vi "Main.vi"() -> ()   [LabVIEW 2017, in "Settings Editor.lvlib"]
doc: "This template is based off of the Queued Message Handler design pattern and the Queued Message Handler project template that ships with LabVIEW.\n\nThe main difference is that the queue is private to this module and communication between modules is performed via Broadcast and Request events.\n\nRequest events are wrapped in public API methods and are handled in the Event Handling Loop (EHL) of this VI. Any module can register for Broadcast events sent by this module. The EHL generates messages based on user interface actions.\n\nThe Message Handling Loop (MHL) processes messages generated by the EHL, or by other messages. The messages are string values, so new messages can be added easily to the Message Cases case structure in the MHL. Each message cluster can also provide an optional value for Message Data, which is a variant that can be converted to whatever message-specific data is required.\n_____\nBased on Delacor QMH Project Template 4.0.0.47.\n_____\nBased on Delacor QMH Project Template 4.1.0.56."
uses:
  Settings Editor.lvlib
  <vilib>/Delacor/Delacor QMH/Libraries/Module Admin_class/Delacor_lib_QMH_Module Admin.lvclass
  CML Shared/Signal Type--enum.ctl
  CML Shared/Calibration Values--cluster.ctl
  Module Data--cluster.ctl
  Settings--cluster.ctl
  Stop Argument--cluster.ctl
  Update Application Settings Argument--cluster.ctl
  Update Application Settings (Reply Payload)--cluster.ctl
  <vilib>/Delacor/Delacor QMH/Libraries/Module Admin_class/Delacor_lib_QMH_Module Admin.lvclass/Delacor_lib_QMH_Module Admin.ctl
  <vilib>/Utility/miscctls.llb/LVPointTypeDef.ctl
  <vilib>/Delacor/Delacor QMH/Libraries/Module Admin_class/Delacor_lib_QMH_Get External Launch.vi
  <vilib>/Delacor/Delacor QMH/Libraries/Message Queue_class/Delacor_lib_QMH_Enqueue Message (Single).vi
  <vilib>/Utility/error.llb/Error Cluster From Error Code.vi
  <vilib>/ErrorRing/Error Ring.xnode
  <vilib>/Delacor/Delacor QMH/Libraries/Message Queue_class/Delacor_lib_QMH_Message Queue.lvclass
  CML Shared/CML Shared.lvlib
panel:
  in  "Calibration Values":T1[](array[typedef])
  in  "Cancel":bool
  in  "OK":bool
  in  "Log File Base Path":path
  in  "Signal Type":T2
  out "error out":errorcluster
  in  "Module Admin":refnum<class "Delacor_lib_QMH_Module Admin.lvclass">
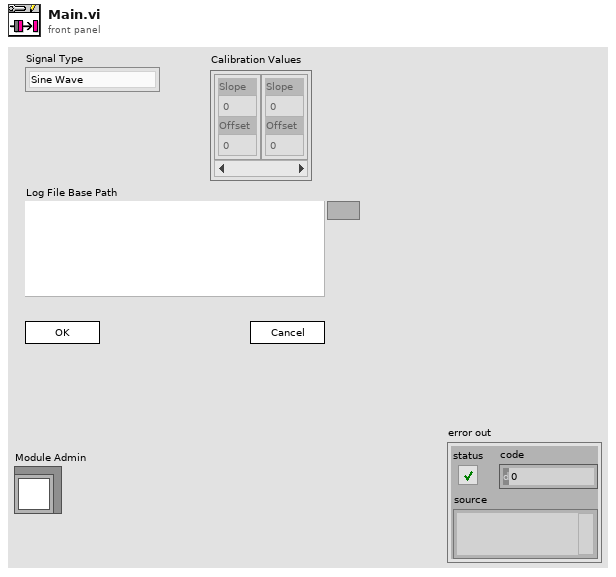
[diagram p1: front panel]
types:
  T1 = typedef "CML Shared.lvlib/Calibration Values--cluster.ctl" = cluster{"Slope":dbl, "Offset":dbl}
  T2 = typedef "CML Shared.lvlib/Signal Type--enum.ctl" = enum16{"Sine Wave", "Square with Noise"}
  T3 = typedef "Settings Editor.lvlib/Request Events--cluster.ctl" = cluster{"Stop Module":refnum<user-event>, "Show Panel":refnum<user-event>, "Hide Panel":refnum<user-event>, "Get Module Execution Status":refnum<user-event>, "Show Diagram":refnum<user-event>, "Update Application Settings":refnum<user-event>}
  T4 = typedef "Settings Editor.lvlib/Module Data--cluster.ctl" = cluster{"Settings":T5}
  T5 = typedef "Settings Editor.lvlib/Settings--cluster.ctl" = cluster{"Signal Type":T2, "Calibration Array":T1[], "Log File Base Path":path}
  T6 = enum32{"invalid lock state", "Not Locked", "Locked (No Password)", "Password-protected"}
  T7 = typedef "Settings Editor.lvlib/Stop Argument--cluster.ctl" = cluster{"Origin":string, "Exit via Stop Module Req?":bool, "Wait for Module to stop?":bool}
  T8 = typedef "Settings Editor.lvlib/Update Application Settings Argument--cluster.ctl" = cluster{"Wait Notifier":refnum<notifier>, "wait for reply":bool}
  T9 = typedef "LVPointTypeDef.ctl" = cluster{"Horizontal":i16, "Vertical":i16}
  T10 = enum32{"Invalid", "Standard", "Closed", "Hidden", "Minimized", "Maximized"}
  T11 = typedef "Settings Editor.lvlib/Update Application Settings (Reply Payload)--cluster.ctl" = cluster{"Settings":T5, "Update Settings_error":errorcluster}
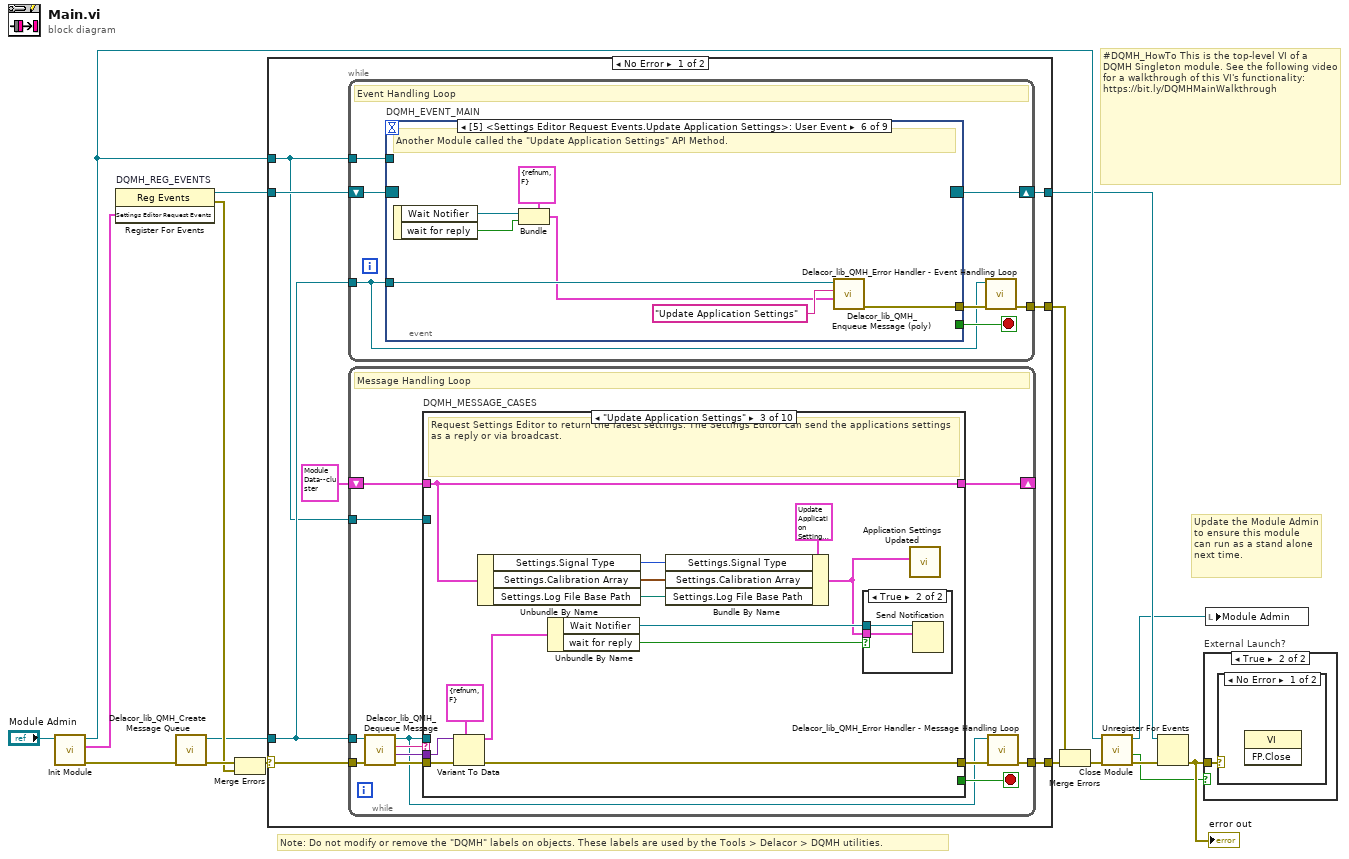
[diagram p0: block diagram]
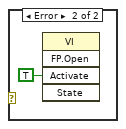
[diagram p3: hidden frame]
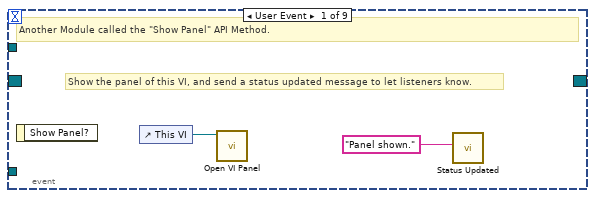
[diagram p4: hidden frame]
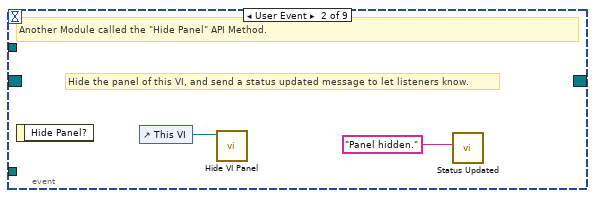
[diagram p5: hidden frame]
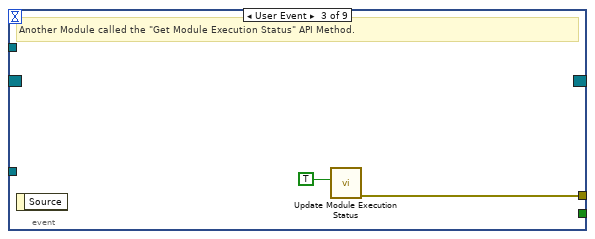
[diagram p6: hidden frame]
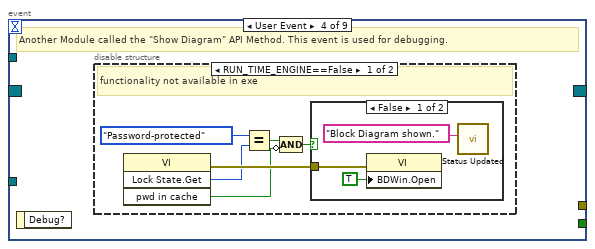
[diagram p7: hidden frame]
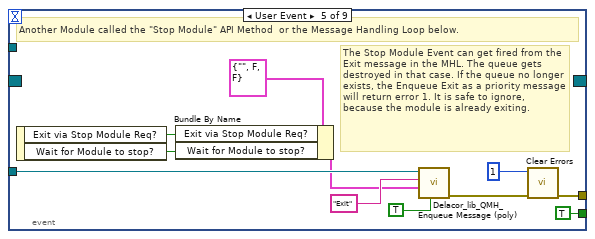
[diagram p10: hidden frame]
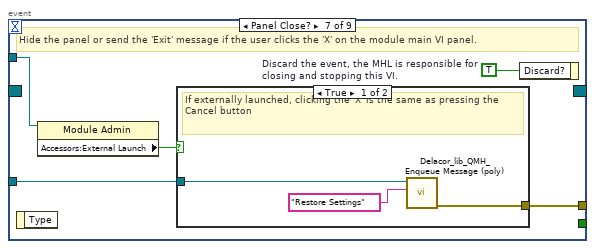
[diagram p11: hidden frame]
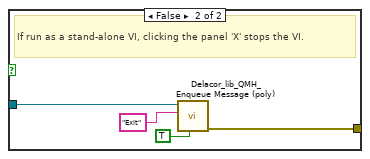
[diagram p12: hidden frame]
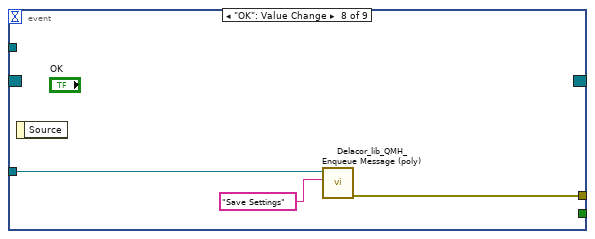
[diagram p13: hidden frame]
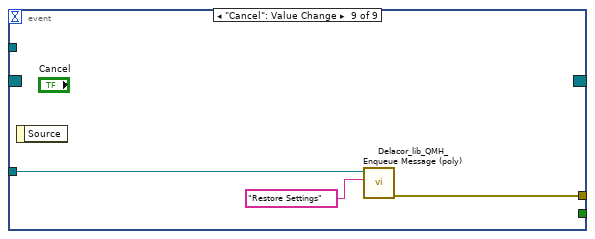
[diagram p14: hidden frame]
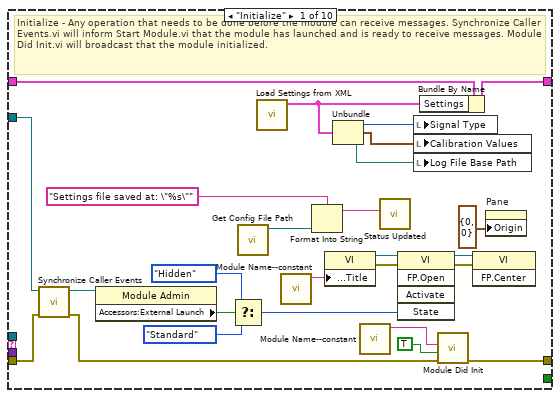
[diagram p15: hidden frame]
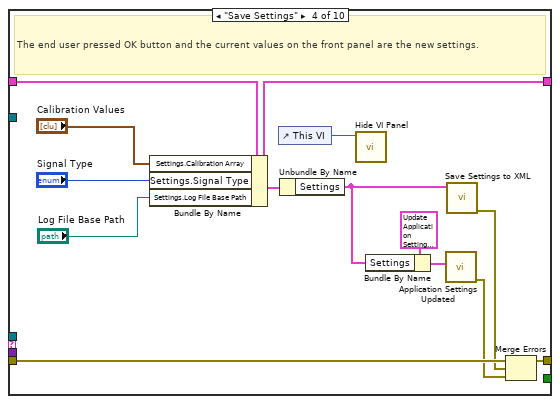
[diagram p18: hidden frame]
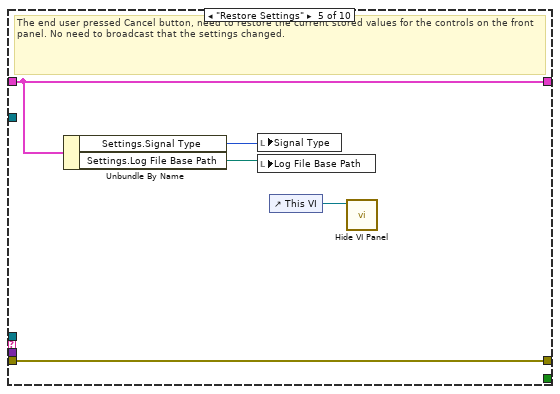
[diagram p19: hidden frame]
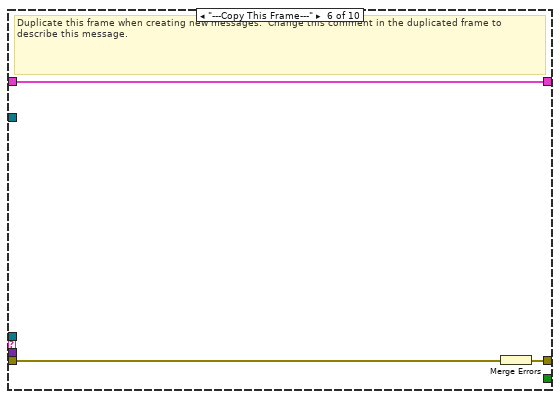
[diagram p20: hidden frame]
diagram:
  # "#DQMH_HowTo This is the top-level VI of a DQMH Singleton module. See the following video for a walkthrough of this VI's functionality: https://bit.ly/DQMHMainWalkthrough"
  # "Note: Do not modify or remove the \"DQMH\" labels on objects. These labels are used by the Tools > Delacor > DQMH utilities."
  # "Update the Module Admin to ensure this module can run as a stand alone next time."
  n1 = call "Init Module.vi"("Singleton Module Admin in"="Module Admin") -> ("error out"=w16:errorcluster, "Settings Editor Request Events"=w5:T3, "Singleton Module Admin out"=w8:refnum<class "Delacor_lib_QMH_Module Admin.lvclass">)  [unwired: 8 in]
  n2 = register-events "DQMH_REG_EVENTS"(w5) -> (reference out=w6:refnum<event-registration>, error out=w9:errorcluster)  [unwired: 2 in]
  n3 = call <vilib>:"Delacor_lib_QMH_Create Message Queue.vi"("error in (no error)"=w16) -> ("error out"=w11:errorcluster, "Message Queue"=w4:refnum<class "Delacor_lib_QMH_Message Queue.lvclass">)  [unwired: 9 in]
  n4 = Merge Errors(w11, w9) -> (w10:errorcluster)
  n5 = case shown="No Error" w10 {
    selector: w10 -> [w23 w214]
    tunnel: [w25 w214] -> w17
    tunnel: [w22 w211] -> w7
    tunnel: w6 -> [w20 w211]
    tunnel: w4 -> [w19 _]
    tunnel: [w24 _] -> w14
    tunnel: w8 -> [w18 w207]
    frame No Error {
      n6 = while {
        tunnel: w19 -> [w26]
        shift-right: [w29] -> w22
        shift-left: w20 -> [w30]
        tunnel: [w31] -> w24
        tunnel: w18 -> [w27]
        stop <- w28 stop-if-true
        # "Event Handling Loop"
        n7 = event "DQMH_EVENT_MAIN" shown="[5] <Settings Editor Request Events.Update Application Settings>: User Event" {
          selector: w30 -> [_ _ _ _ _ _ _ _ _]
          dyn-events: [_ _ _ _ _ _ _ _ _] -> w29
          timeout: _ -> [_ _ _ _ _ _ _ _ _]
          tunnel: [_ _ _ _ TRUE ("Discard?") _ _ _ _] -> w28
          tunnel: w26 -> [_ _ _ _ w54 w65 w68 w78 w82]
          tunnel: [_ _ w38 _ w57 w61 w70 w79 w81] -> w32
          tunnel: w27 -> [_ _ _ _ _ _ w67 _ _]
          event User Event {
            # "Show the panel of this VI, and send a status updated message to let listeners know."
            # "Another Module called the \"Show Panel\" API Method."
            n8 = event-data() -> ()  [unwired: 1 in, 1 out]
            n9 = control-ref of="This VI"() -> (w34:refnum<vi>)
            n10 = call "Open VI Panel.vi"("VI"=w34) -> ()  [unwired: 10 in, 1 out]
            n11 = call "Status Updated.vi"("Status"="Panel shown." ("format string")) -> ()  [unwired: 10 in, 1 out]
          }
          event User Event {
            # "Hide the panel of this VI, and send a status updated message to let listeners know."
            # "Another Module called the \"Hide Panel\" API Method."
            n12 = event-data() -> ()  [unwired: 1 in, 1 out]
            n13 = control-ref of="This VI"() -> (w36:refnum<vi>)
            n14 = call "Hide VI Panel.vi"("VI"=w36) -> ()  [unwired: 10 in, 1 out]
            n15 = call "Status Updated.vi"("Status"="Panel hidden." ("format string")) -> ()  [unwired: 10 in, 1 out]
          }
          event User Event {
            # "Another Module called the \"Get Module Execution Status\" API Method."
            n16 = event-data() -> ()  [unwired: 1 in, 1 out]
            n17 = call "Update Module Execution Status.vi"("Running?"=TRUE) -> ("error out"=w38:errorcluster)  [unwired: 10 in]
          }
          event User Event {
            # "Another Module called the \"Show Diagram\" API Method. This event is used for debugging."
            n18 = event-data() -> ()  [unwired: 1 in, 1 out]
            n19 = disable-structure shown="RUN_TIME_ENGINE==False" {
              frame condition #0 (active) {
                # "functionality not available in exe"
                n20 = invoke class="VI" method="Lock State.Get"() -> (error out=w44:errorcluster, "Get Lock State"=w43:T6, "pwd in cache"=w40:bool)  [unwired: 4 in, 1 out]
                n21 = Equal?(x=T6."Password-protected", y=w43) -> (x = y?=w41:bool)
                n22 = Compound Arithmetic op=AND(w41, invert w40) -> (w39:bool)
                n23 = case shown="False" w39 {
                  tunnel: w44 -> [w47 _]
                  frame False {
                    n24 = property class="VI"(error in=w47, "BDWin.Open"=TRUE ("Block Diagram Window:Open")) -> ()  [unwired: 1 in, 2 out]
                    n25 = call "Status Updated.vi"("Status"="Block Diagram shown." ("format string")) -> ()  [unwired: 10 in, 1 out]
                  }
                  frame True {
                    # "Password-protected VI, and the password is not in the cache. Do not show the diagram."
                  }
                }
              }
              frame condition #1 {
              }
            }
          }
          event User Event {
            # "The Stop Module Event can get fired from the Exit message in the MHL. The queue gets destroyed in that case. If the queue no longer exists, the Enqueue Exit as a priority message will return error 1. It is safe to ignore, because the module is already exiting."
            # "Another Module called the \"Stop Module\" API Method  or the Message Handling Loop below."
            n26 = event-data() -> ("Exit via Stop Module Req?"=w50:bool, "Wait for Module to stop?"=w49:bool)  [unwired: 1 in]
            n27 = Bundle By Name(cluster=T7 {"Origin"="", "Exit via Stop Module Req?"=FALSE, "Wait for Module to stop?"=FALSE} ("Stop Argument"), "Exit via Stop Module Req?"=w50, "Wait for Module to stop?"=w49) -> (w48:T7)
            n28 = call-poly <vilib>:"Delacor_lib_QMH_Enqueue Message (poly).vi"("Priority Message? (F)"=TRUE, "Message Data"=w48, "Message"="Exit", "Message Queue in"=w54) -> ("error out"=w58:errorcluster)  [unwired: 6 in, 1 out]
            n29 = call <vilib>:"Clear Errors.vi"("error in (no error)"=w58, "specific error code to clear (0: all)"=1) -> ("error out"=w57:errorcluster)  [unwired: 4 in, 1 out]
          }
          event User Event {
            # "Another Module called the \"Update Application Settings\" API Method."
            n30 = event-data() -> ("Wait Notifier"=w60:refnum<notifier>, "wait for reply"=w59:bool)  [unwired: 1 in]
            n31 = Bundle(cluster=T8 {"Wait Notifier"=refnum, "wait for reply"=FALSE} ("Update Application Settings Argument"), "Wait Notifier"=w60, "wait for reply"=w59) -> (w62:T8)
            n32 = call-poly <vilib>:"Delacor_lib_QMH_Enqueue Message (poly).vi"("Message Data"=w62, "Message"="Update Application Settings", "Message Queue in"=w65) -> ("error out"=w61:errorcluster)  [unwired: 7 in, 1 out]
          }
          event Panel Close? {
            w69 = TRUE  # Discard the event, the MHL is responsible for closing and stopping this VI.
            # "Hide the panel or send the 'Exit' message if the user clicks the 'X' on the module main VI panel."
            n33 = event-data() -> ()  [unwired: 1 in, 1 out]
            n34 = property class="Module Admin"(reference=w67) -> ("Accessors:External Launch"=w66:bool)  [unwired: 1 in, 2 out]
            n35 = case shown="True" w66 {
              tunnel: w68 -> [w72 w76]
              tunnel: [w71 w77] -> w70
              frame True {
                # "If externally launched, clicking the 'X' is the same as pressing the Cancel button"
                n36 = call-poly <vilib>:"Delacor_lib_QMH_Enqueue Message (poly).vi"("Message"="Restore Settings", "Message Queue in"=w72) -> ("error out"=w71:errorcluster)  [unwired: 8 in, 1 out]
              }
              frame False {
                # "If run as a stand-alone VI, clicking the panel 'X' stops the VI."
                n37 = call-poly <vilib>:"Delacor_lib_QMH_Enqueue Message (poly).vi"("Priority Message? (F)"=TRUE, "Message"="Exit", "Message Queue in"=w76) -> ("error out"=w77:errorcluster)  [unwired: 7 in, 1 out]
              }
            }
            n38 = event-data("Discard?"=w69) -> ()  [unwired: 1 in, 1 out]
          }
          event "OK": Value Change {
            n39 = event-data() -> ()  [unwired: 1 in, 1 out]
            n40 = call-poly <vilib>:"Delacor_lib_QMH_Enqueue Message (poly).vi"("Message"="Save Settings", "Message Queue in"=w78) -> ("error out"=w79:errorcluster)  [unwired: 8 in, 1 out]
          }
          event "Cancel": Value Change {
            n41 = event-data() -> ()  [unwired: 1 in, 1 out]
            n42 = call-poly <vilib>:"Delacor_lib_QMH_Enqueue Message (poly).vi"("Message"="Restore Settings", "Message Queue in"=w82) -> ("error out"=w81:errorcluster)  [unwired: 8 in, 1 out]
          }
        }
        n43 = call-dynamic "Delacor_lib_QMH_Error Handler - Event Handling Loop.vi"("error in (no error)"=w32, "Message Queue in"=w26) -> ("dup error in"=w31:errorcluster)  [unwired: 8 in, 1 out]
      }
      n44 = while {
        tunnel: w19 -> [w86]
        shift-right: [w90] -> _
        shift-left: T4 {"Settings"={"Signal Type"=enum."Sine Wave", "Calibration Array"=[{"Slope"=1.0, "Offset"=0.0}], "Log File Base Path"=path ""}} ("Data Cluster") -> [w91]
        tunnel: w23 -> [w94]
        tunnel: [w92] -> w25
        tunnel: w18 -> [w84]
        stop <- w89 stop-if-true
        # "Message Handling Loop"
        n45 = call-dynamic "Delacor_lib_QMH_Dequeue Message.vi"("error in (no error)"=w94, "Message Queue in"=w86) -> ("error out"=w93:errorcluster, "Message Data"=w87:variant, "Message"=w88:string, "Message Queue out"=w85:refnum<class "Delacor_lib_QMH_Message Queue.lvclass">)  [unwired: 6 in]
        n46 = case "DQMH_MESSAGE_CASES" shown="\"Update Application Settings\"" w88 {
          selector: w88 -> [_ _ _ _ _ _ _ _ _ w194]
          tunnel: w85 -> [_ _ _ _ _ _ _ w164 w186 _]
          tunnel: w93 -> [w120 w123 w136 w141 w156 w159 w161 w171 w192 w196]
          tunnel: [w118 w123 w135 w142 w156 w158 w161 w167 w189 w197] -> w95
          tunnel: w91 -> [w109 w122 w129 w151 w155 w157 w160 w166 w185 w195]
          tunnel: [w108 w122 w129 w148 w155 w157 w160 w166 w185 w195] -> w90
          tunnel: [_ _ _ _ _ _ _ _ w184 _] -> w89
          tunnel: w87 -> [_ _ w134 _ _ _ _ w165 w183 _]
          tunnel: w84 -> [w110 _ _ _ _ _ _ w163 w178 _]
          frame "Initialize" {
            # "Initialize - Any operation that needs to be done before the module can receive messages. Synchronize Caller Events.vi will inform Start Module.vi that the module has launched and is ready to receive messages. Module Did Init.vi will broadcast that the module initialized."
            n47 = call "Synchronize Caller Events.vi"("error in (no error)"=w120, "Singleton Module Admin in"=w110) -> ("error out"=w119:errorcluster, "Singleton Module Admin out"=w105:refnum<class "Delacor_lib_QMH_Module Admin.lvclass">)  [unwired: 8 in]
            n48 = property class="Module Admin"(reference=w105) -> ("Accessors:External Launch"=w114:bool)  [unwired: 1 in, 2 out]
            n49 = Select(t=T10."Hidden" ("State"), s=w114, f=T10."Standard" ("State")) -> (s? t:f=w111:T10)
            n50 = call "Get Config File Path.vi"() -> ("XML File Path"=w102:path)  [unwired: 10 in, 1 out]
            n51 = call "Load Settings from XML.vi"() -> ("Settings out"=w99:T5)  [unwired: 10 in, 1 out]
            n52 = call "Module Name--constant.vi"() -> ("Module Name"=w117:string)  [unwired: 11 in]
            n53 = Format Into String(format string="Settings file saved at: \"%s\"", w102) -> (resulting string=w101:string)  [unwired: 2 in, 1 out]
            n54 = property class="VI"("Front Panel.Title"=w117) -> (reference out=w116:refnum<vi>, error out=w103:errorcluster)  [unwired: 2 in]
            n55 = Unbundle(w99) -> ("Signal Type"=w98:T2, "Calibration Array"=w97:T1[], "Log File Base Path"=w96:path)
            n56 = call "Module Name--constant.vi"() -> ("Module Name"=w106:string)  [unwired: 11 in]
            n57 = call "Status Updated.vi"("Status"=w101) -> ()  [unwired: 10 in, 1 out]
            n58 = invoke class="VI" method="FP.Open"(reference=w116, error in=w103, "State"=w111) -> (reference out=w115:refnum<vi>, error out=w121:errorcluster)  [unwired: 2 in, 3 out]
            n59 = local write "Signal Type"(w98) -> ()
            n60 = local write "Calibration Values"(w97) -> ()
            n61 = local write "Log File Base Path"(w96) -> ()
            n62 = Bundle By Name(cluster=w109, "Settings"=w99) -> (w108:T4)
            n63 = call "Module Did Init.vi"("error in (no error)"=w119, "Initialized?"=TRUE, "Origin"=w106) -> ("error out"=w118:errorcluster)  [unwired: 8 in]
            n64 = invoke class="VI" method="FP.Center"(reference=w115, error in=w121) -> ()  [unwired: 1 in, 3 out]
            n65 = property on="Pane" class="Pane"("Origin"=T9 {"Horizontal"=0, "Vertical"=0}) -> ()  [unwired: 2 in, 2 out]
          }
          frame "--- Module Specific ---" {
            # "Separator -- The following cases handle messages specific to this Module."
          }
          frame "Update Application Settings" {
            # "Request Settings Editor to return the latest settings. The Settings Editor can send the applications settings as a reply or via broadcast."
            n66 = Variant To Data(error in=w136, type=T8 {"Wait Notifier"=refnum, "wait for reply"=FALSE} ("Update Application Settings Argument"), Variant=w134) -> (data=w132:T8, error out=w135:errorcluster)
            n67 = Unbundle By Name(w129) -> ("Settings.Signal Type"=w127:T2, "Settings.Calibration Array"=w126:T1[], "Settings.Log File Base Path"=w125:path)
            n68 = Unbundle By Name(w132) -> ("Wait Notifier"=w131:refnum<notifier>, "wait for reply"=w130:bool)
            n69 = Bundle By Name(cluster=T11 {"Settings"={"Signal Type"=enum."Sine Wave", "Calibration Array"=[], "Log File Base Path"=path ""}, "Update Settings_error"={"status"=FALSE, "code"=0, "source"=""}} ("Update Application Settings (Reply Payload)"), "Settings.Signal Type"=w127, "Settings.Calibration Array"=w126, "Settings.Log File Base Path"=w125) -> (w124:T11)
            n70 = case shown="True" w130 {
              tunnel: w131 -> [_ w138]
              tunnel: w124 -> [_ w137]
              frame False {
              }
              frame True {
                n71 = Send Notification(notification=w137, notifier=w138) -> ()  [unwired: 1 in, 2 out]
              }
            }
            n72 = call "Application Settings Updated.vi"("Reply Payload"=w124) -> ()  [unwired: 10 in, 1 out]
          }
          frame "Save Settings" {
            # "The end user pressed OK button and the current values on the front panel are the new settings."
            n73 = Bundle By Name(cluster=w151, "Settings.Calibration Array"="Calibration Values", "Settings.Signal Type"="Signal Type", "Settings.Log File Base Path"="Log File Base Path") -> (w148:T4)
            n74 = control-ref of="This VI"() -> (w149:refnum<vi>)
            n75 = Unbundle By Name(w148) -> ("Settings"=w143:T5)
            n76 = call "Hide VI Panel.vi"("VI"=w149) -> ()  [unwired: 10 in, 1 out]
            n77 = Bundle By Name(cluster=T11 {"Settings"={"Signal Type"=enum."Sine Wave", "Calibration Array"=[], "Log File Base Path"=path ""}, "Update Settings_error"={"status"=FALSE, "code"=0, "source"=""}} ("Reply Payload"), "Settings"=w143) -> (w144:T11)
            n78 = call "Application Settings Updated.vi"("Reply Payload"=w144) -> ("error out"=w139:errorcluster)  [unwired: 10 in]
            n79 = call "Save Settings to XML.vi"("Settings"=w143) -> ("error out"=w140:errorcluster)  [unwired: 10 in]
            n80 = Merge Errors(w141, w140, w139) -> (w142:errorcluster)
          }
          frame "Restore Settings" {
            # "The end user pressed Cancel button, need to restore the current stored values for the controls on the front panel. No need to broadcast that the settings changed."
            n81 = Unbundle By Name(w155) -> ("Settings.Signal Type"=w154:T2, "Settings.Log File Base Path"=w153:path)
            n82 = local write "Signal Type"(w154) -> ()
            n83 = local write "Log File Base Path"(w153) -> ()
            n84 = control-ref of="This VI"() -> (w152:refnum<vi>)
            n85 = call "Hide VI Panel.vi"("VI"=w152) -> ()  [unwired: 10 in, 1 out]
          }
          frame "---Copy This Frame---" {
            # "Duplicate this frame when creating new messages.  Change this comment in the duplicated frame to describe this message."
            n86 = Merge Errors(w159) -> (w158:errorcluster)
          }
          frame "--- Exit and Error Handling---" {
            # "Separator - The following cases handle errors and exit messages."
          }
          frame "Error" {
            # "#CodeRecommended - If you ever change the name of this \"Error\" message, you'll need to update the name in the Check Loop Error.vi as well."
            # "#CodeRecommended - If the module is running in standalone mode (External Launch = FALSE), this code will pop up an error dialog and call the 'Exit' message if an error occurs. Add more fine-grained error handling here."
            # "Error - Check the error message data and respond accordingly. This message is sent by the \"Error Handler\" VIs at the end of each loop in this application."
            n87 = property class="Module Admin"(reference=w163) -> ("Accessors:External Launch"=w162:bool)  [unwired: 1 in, 2 out]
            n88 = Variant To Data(error in=w171, type=errorcluster {"status"=FALSE, "code"=0, "source"=""} ("error constant"), Variant=w165) -> (data=w172:errorcluster, error out=w169:errorcluster)
            n89 = call "Error Reported.vi"("Error"=w172) -> ()  [unwired: 10 in, 1 out]
            n90 = case shown="False" w162 {
              tunnel: [w177 _] -> w168
              tunnel: w164 -> [w175 _]
              tunnel: w172 -> [w176 _]
              frame False {
                # "If the module is running standalone, then pop up an error dialog and call the \"Exit\" message."
                n91 = call <vilib>:"Simple Error Handler.vi"("error in (no error)"=w176) -> ()  [unwired: 4 in, 5 out]
                n92 = call-poly <vilib>:"Delacor_lib_QMH_Enqueue Message (poly).vi"("Priority Message? (F)"=TRUE, "Message"="Exit", "Message Queue in"=w175) -> ("error out"=w177:errorcluster)  [unwired: 7 in, 1 out]
              }
              frame True {
                # "If the module was launched externally, calling the Error Reported broadcast VI is the only action performed by the \"Error\" message. The module's caller can then process the error appropriately."
              }
            }
            n93 = Merge Errors(w169, w168) -> (w167:errorcluster)
            n94 = local write "error out"(w167) -> ()
          }
          frame "Exit" {
            w182 = 91  # 91: not all Exit messages will have an argument
            w184 = TRUE  # Stop the VI
            # "Release the message queue reference"
            # "#CodeNeeded - Add any required cleanup code here"
            # "Exit - Exit the application."
            n95 = Variant To Data(error in=w192, type=T7 {"Origin"="", "Exit via Stop Module Req?"=FALSE, "Wait for Module to stop?"=FALSE} ("Stop Argument"), Variant=w183) -> (data=w180:T7, error out=w188:errorcluster)
            n96 = call <vilib>:"Clear Errors.vi"("error in (no error)"=w188, "specific error code to clear (0: all)"=w182) -> ("error out"=w191:errorcluster)  [unwired: 4 in, 1 out]
            n97 = control-ref of="This VI"() -> (w179:refnum<vi>)
            n98 = call-dynamic "Delacor_lib_QMH_Release Message Queue.vi"("error in (no error)"=w191, "Message Queue"=w186) -> ("error out"=w190:errorcluster)  [unwired: 9 in]
            n99 = call "Handle Exit.vi"("Stop Argument"=w180, "Admin in"=w178, "VI reference"=w179) -> ("error out"=w187:errorcluster)  [unwired: 7 in, 1 out]
            n100 = Merge Errors(w190, w187) -> (w189:errorcluster)
          }
          frame Default {
            # "'Default' case only runs if there is a message that isn't defined in any of the other cases.  Output a programming error."
            n101 = call "Module Name--constant.vi"() -> ("Module Name"=w193:string)  [unwired: 11 in]
            n102 = xnode "Error Ring"("parameter 0"=w194, "parameter 1"=w193) -> ("error out"=w198:errorcluster)
            n103 = Merge Errors(w196, w198) -> (w197:errorcluster)
          }
        }
        n104 = call-dynamic "Delacor_lib_QMH_Error Handler - Message Handling Loop.vi"("error in (no error)"=w95, "Message Queue in"=w85) -> ("dup error in"=w92:errorcluster)  [unwired: 8 in, 1 out]
      }
    }
    frame Error {
      # "Synchronize Caller Events.vi will inform Start Module.vi that the module has launched and will let the code calling Start Module.vi register for broadcasts and would permit the caller receive the broadcast that an error occurred at launch time."
      n105 = call "Synchronize Caller Events.vi"("Singleton Module Admin in"=w207) -> ("error out"=w212:errorcluster)  [unwired: 9 in, 1 out]
      n106 = call "Module Name--constant.vi"() -> ("Module Name"=w210:string)  [unwired: 11 in]
      n107 = Format Into String(format string="An error occurred during initialization. %s is no longer running.", w210) -> (resulting string=w208:string)  [unwired: 2 in, 1 out]
      n108 = Merge Errors(w214, w212) -> (w213:errorcluster)
      n109 = call "Error Reported.vi"("Additional Information"=w208, "Error"=w213) -> ()  [unwired: 9 in, 1 out]
    }
  }
  n110 = Merge Errors(w14, w17) -> (w13:errorcluster)
  n111 = call "Close Module.vi"("error in (no error)"=w13, "Module Admin in"=w8) -> ("error out"=w15:errorcluster, "External Launch"=w1:bool, "Module Admin out"=w2:refnum<class "Delacor_lib_QMH_Module Admin.lvclass">)  [unwired: 7 in]
  n112 = Unregister For Events(event registration refnum=w7, error in=w15) -> (error out=w12:errorcluster)
  "error out" <- w12
  n113 = case "External Launch?" shown="True" w1 {
    tunnel: w12 -> [_ w215]
    frame False {
    }
    frame True {
      n114 = case shown="No Error" w215 {
        frame No Error {
          n115 = invoke class="VI" method="FP.Close"() -> ()  [unwired: 3 in, 3 out]
        }
        frame Error {
          n116 = invoke class="VI" method="FP.Open"("Activate"=TRUE ("Activate?")) -> ()  [unwired: 4 in, 5 out]
        }
      }
    }
  }
  n117 = local write "Module Admin"(w2) -> ()
